vi "Get Item GUID.vi"(8 "error in (no error)":errorcluster, 11 "item in":T1 format="%.0x") -> (0 "error out":errorcluster, 2 "guid":string, 3 "item out":T1 format="%.0x")   [LabVIEW 2020, in "XNET System Explorer.lvlib"]
uses:
  XNET System Explorer.lvlib
  NationalInstruments.VeriStand.SystemDefinitionAPI
  <vilib>/NI VeriStand/Custom Device API/Custom Device Item Ref.ctl
  <vilib>/NI VeriStand/Custom Device API/Custom Device API.lvlib
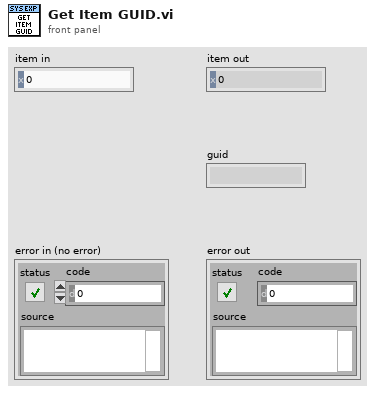
[diagram p1: front panel]
types:
  T1 = typedef "Custom Device API.lvlib/Custom Device Item Ref.ctl" = u64
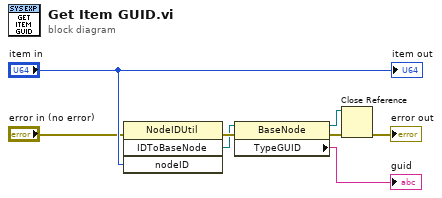
[diagram p0: block diagram]
diagram:
  n1 = invoke class="NodeIDUtil" method="IDToBaseNode"(error in="error in (no error)", "nodeID"="item in") -> (error out=w3:errorcluster, "IDToBaseNode"=w2:refnum<k24>)  [unwired: 2 in, 2 out]
  n2 = property class="BaseNode"(reference=w2, error in=w3) -> (reference out=w5:refnum<k24>, error out=w4:errorcluster, "TypeGUID"=→"guid":string)
  n3 = Close Reference(reference=w5, error in (no error)=w4) -> (error out=→"error out":errorcluster)
  "item out" <- "item in"
